vi "Test error after assertion.vi"(8 "error in (no error)":errorcluster, 11 "TestCase in":refnum<class "VI Test Comparison.lvclass">) -> (0 "error out":errorcluster, 3 "TestCase out":refnum<class "VI Test Comparison.lvclass">)   [LabVIEW 2020, in "VI Test Comparison.lvclass"]
uses:
  VI Test Comparison.lvclass
  <vilib>/addons/_JKI Toolkits/VI Tester/TestCase.llb/TestCase.lvclass
  C:/Program Files (x86)/National Instruments/LabVIEW 2020/vi.lib/addons/_JKI Toolkits/VI Tester/TestCase.llb/TestCase.lvclass
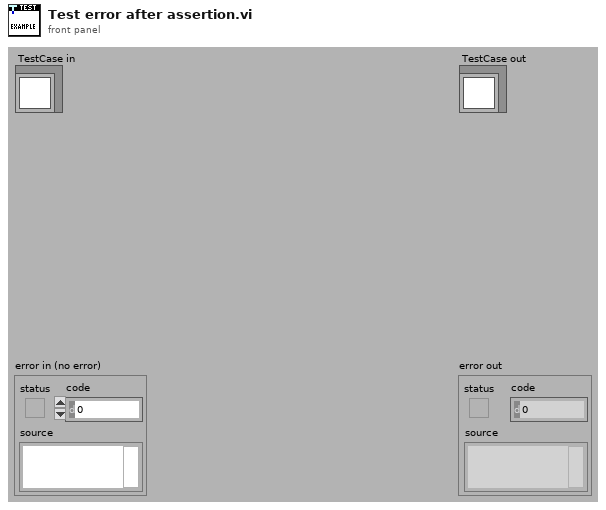
[diagram p1: front panel]
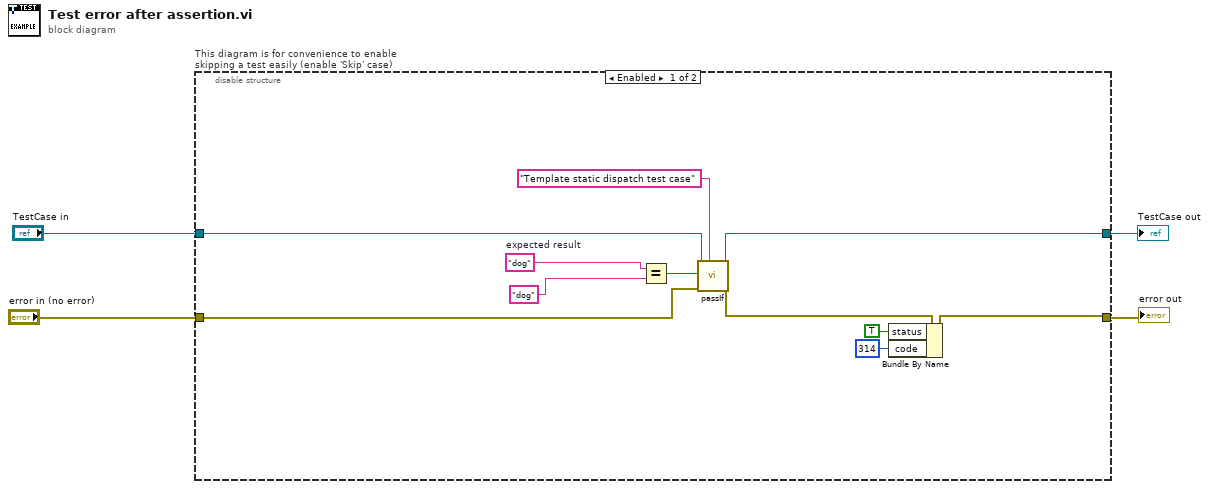
[diagram p0: block diagram]
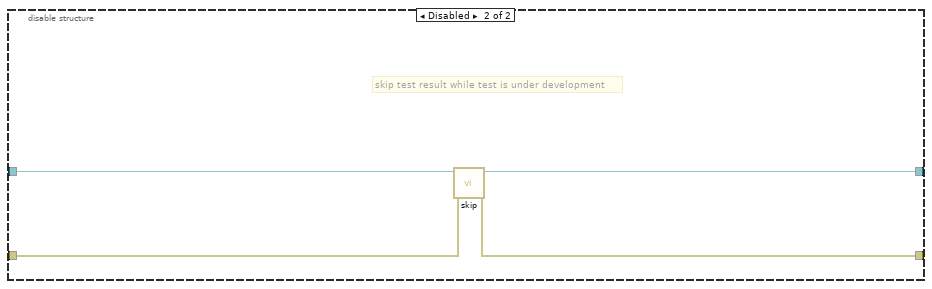
[diagram p2: hidden frame]
diagram:
  n1 = disable-structure "This diagram is for convenience to enable skipping a test easily (enable 'Skip' case)" shown="Enabled" {
    disable-tunnel: "TestCase in" -> [w15 w19]
    disable-tunnel: [w14 w17] -> w1
    disable-tunnel: [w11 w18] -> w3
    disable-tunnel: "error in (no error)" -> [w12 w16]
    frame Enabled {
      w6 = "dog"  # expected result
      n2 = Equal?(x=w6, y="dog" ("expected result")) -> (x = y?=w5:bool)
      n3 = call-dynamic "passIf.vi"("custom report message (\"\")"="Template static dispatch test case" ("Description"), "error in (no error)"=w12, "pass"=w5, "TestCase in"=w15) -> ("error out"=w13:errorcluster, "TestCase out"=w14:refnum<class "VI Test Comparison.lvclass">)  [unwired: 6 in]
      n4 = Bundle By Name(cluster=w13, "status"=TRUE, "code"=314) -> (w11:errorcluster)
    }
    frame Disabled {
      # "skip test result while test is under development"
      n5 = call <vilib>:"skip.vi"("error in (no error)"=w16, "TestCase in"=w19) -> ("error out"=w18:errorcluster, "TestCase out"=w17:refnum<class "VI Test Comparison.lvclass">)  [unwired: 8 in]
    }
  }
  "error out" <- w3
  "TestCase out" <- w1
